vi "Gage-Transfer.vi"(4 "Length (4096)":dbl=4096.0, 5 "Start (0)":dbl, 6 "Segment (1)":u32=1, 7 "Mode (0)":u32 step=1, 8 "Channel (0)":u16 step=1, 9 "Handle Cluster":T1) -> (0 "Error Code":i32, 1 "Actual Length":dbl, 2 "Data in Volts":dbl[](array[numeric]) format="%.2f", 3 "Actual Start":dbl)   [LabVIEW 2022 SP3]
doc: "This VI transfers the data from one channel of the CompuScope system identified by Handle Cluster, which is obtained by calling CsTool-GetSystem.vi. For accurate interpretation of the transferred data, the user should always use the returned Actual Start and Actual Length, and not the requested values. \n\nThis VI can be used for transferring data from 8, 12, 14, and 16 bit CompuScope hardware. Data are transferred from on-board CompuScope memory to PC RAM using PCI Bus Mastering at rates of up to 200 MB/s. \n\nInternally, CsTool-Transfer.vi converts the raw integer ADC code values into double variable voltage values. For more rapid data access, the user may remove the voltage conversion step. The VI will not return programmatic control to LabVIEW until all of the data have been transferred. \n\nIf the call is successful, a 1 is returned in the Error Code indicator. If the call is unsuccessful, an appropriate error code is returned. A descriptive error string may be obtained by calling CsTool-ErrorHandler.vi.\n\n\nInput Value Descriptions:\n\nChannel\nThis integer value specifies the channel from which data are to be transferred. The default value is 0 for the first channel in the CompuScope system. Channels in a LabVIEW CompuScope system begin at 0. If an invalid channel number is given, an error will be returned. Please see the CompuScope hardware manual for more information on channel enumeration.\n\nMode\nThis integer value determines the current transfer mode. Currently, the only valid value for this input is 0.\n\nSegment(1)\nThis integer value determines which Multiple Record segment is to be transferred, if the CompuScope hardware was operating in Multiple Record Mode. For Single Record Mode acquisitions, the user must always set the Record value to 1, which is the default value. If the Record value is too large, an error code will be returned. \n\nStart\nThis double variable value determines the requested starting point of the data transfer from CompuScope memory to PC RAM. Start is specified relative to the trigger address for the acquisition. A Start value of 0 will cause data transfer to begin at the trigger address. Negative Start values are used for the transfer of pre-trigger data. Positive Start values may be used to begin transfer after the trigger address. The default Start value is 0. \n\nLength\nThis double variable value specifies the amount of data, in samples, to be transferred. The default value is 4096. \n\nData in Volts\nThis array variable, of type double, is the LabVIEW buffer variable into which transferred data are returned. The size of the array will be at least Length samples. Data are returned as voltage values, whose conversion depends upon the resolution of the CompuScope system and on the current input range.\n\nActual Start\nThis double variable value returns the actual start point of the data array. The Actual Start may be lower than the requested Start value. This is because the CompuScope memory architecture may force the drivers to download data from an earlier point than the start position. For example, if Start is input to CsTool-Transfer.vi as 0, the Actual Start may return as -2, indicating that two extra samples were returned before the Start position. \n\nThe user must account for the discrepancy between the Start and the Actual Start. The user may choose to ignore samples transferred from before the Start position. Alternatively, the user may conserve these samples, accounting for the fact that the values begin at Actual Start. \n\nActual Length\nThis double variable value returns the actual amount of data transferred, which may be different from the requested Length. The difference, if any, results from CompuScope memory architecture."
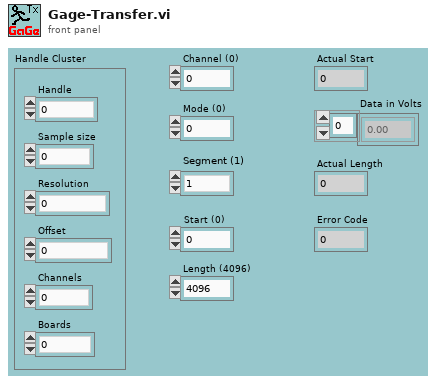
[diagram p1: front panel]
types:
  T1 = cluster{"Handle":u32, "Sample size":u32, "Resolution":i32, "Offset":i32, "Channels":u32, "Boards":u32}
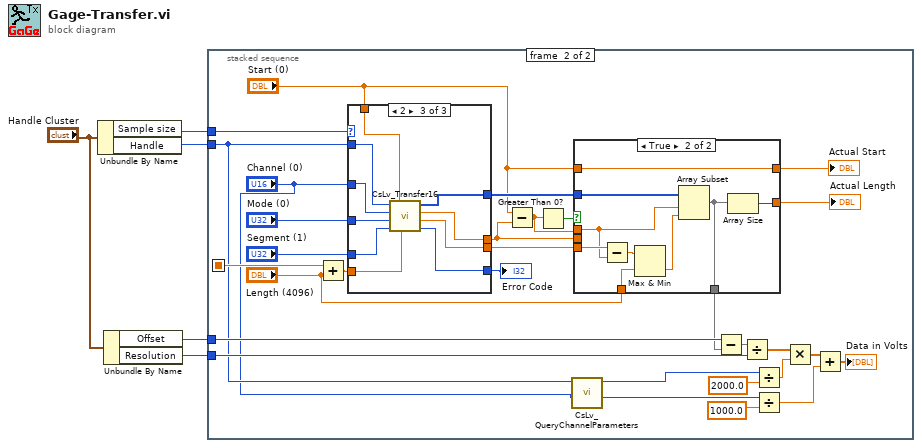
[diagram p0: block diagram]
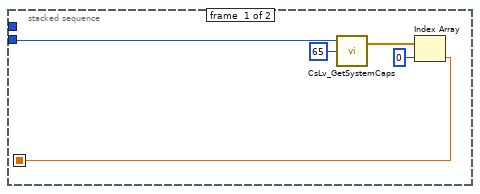
[diagram p2: hidden frame]
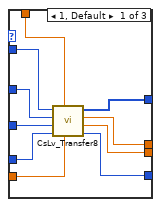
[diagram p4: hidden frame]
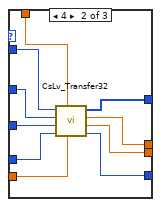
[diagram p5: hidden frame]
diagram:
  n1 = Unbundle By Name("Handle Cluster") -> ("Sample size"=w5:u32, "Handle"=w2:u32)
  n2 = Unbundle By Name("Handle Cluster") -> ("Offset"=w3:i32, "Resolution"=w1:i32)
  n3 = stacked-sequence {
    seq-local: [w6 _] -> [_ w13]
    tunnel: w5 -> [_ w36]
    tunnel: w3 -> [_ w19]
    tunnel: w2 -> [w7 w12]
    tunnel: w1 -> [_ w16]
    frame #0 {
      n4 = call <userlib>:"CsLv_GetSystemCaps.vi"("CapsID"=u16 65, "Handle"=w7) -> ("Buffer"=w9:dbl[])  [unwired: 1 in, 1 out]
      n5 = Index Array(array=w9, index=0) -> (element=w6:dbl)
    }
    frame #1 {
      n6 = Add(x=w13, y="Length (4096)") -> (x+y=w15:dbl)
      n7 = case shown="2" w36 {
        tunnel: w15 -> [w62 w69 w82]
        tunnel: "Segment (1)" -> [w55 w70 w75]
        tunnel: "Mode (0)" -> [w54 w71 w74]
        tunnel: "Start (0)" -> [w61 w68 w81]
        tunnel: [w60 w64 w80] -> w21
        tunnel: [w59 w65 w79] -> w38
        tunnel: [w58 w67 w78] -> w25
        tunnel: w12 -> [w57 w72 w77]
        tunnel: [w56 w66 w76] -> w23
        tunnel: "Channel (0)" -> [w53 w63 w73]
        frame 1, Default {
          n8 = call <userlib>:"CsLv_Transfer8.vi"("Length (4096)"=w62, "Start (0)"=w61, "Segment (1)"=w55, "Mode (0)"=w54, "Channel (0)"=w53, "Handle"=w57) -> ("Error Code"=w59:i32, "Actual Length"=w60:dbl, "Actual Start"=w56:dbl, "Buffer"=w58:u8[])
        }
        frame 4 {
          n9 = call <userlib>:"CsLv_Transfer32.vi"("Length (4096)"=w69, "Start (0)"=w68, "Segment (1)"=w70, "Mode (16)"=w71, "Channel (0)"=w63, "Handle"=w72) -> ("Error Code"=w65:i32, "Actual Length"=w64:dbl, "Actual Start"=w66:dbl, "Buffer"=w67:i32[])
        }
        frame 2 {
          n10 = call <userlib>:"CsLv_Transfer16.vi"("Length (4096)"=w82, "Start (0)"=w81, "Segment (1)"=w75, "Mode (0)"=w74, "Channel (0)"=w73, "Handle"=w77) -> ("Error Code"=w79:i32, "Actual Length"=w80:dbl, "Actual Start"=w76:dbl, "Buffer"=w78:i16[])
        }
      }
      "Error Code" <- w38
      n11 = Subtract(x="Start (0)", y=w23) -> (x-y=w26:dbl)
      n12 = Greater Than 0?(x=w26) -> (x > 0?=w27:bool)
      n13 = call <userlib>:"CsLv_QueryChannelParameters.vi"("Channel"="Channel (0)", "Handle"=w12) -> ("DC Offset (mV)"=w32:i32, "Input Range (mV)"=w31:u32)  [unwired: 5 out]
      n14 = case shown="True" w27 {
        tunnel: w26 -> [_ w49]
        tunnel: [w41 w52] -> w18
        tunnel: w21 -> [w43 w50]
        tunnel: [w43 w51] -> w20
        tunnel: "Length (4096)" -> [_ w46]
        tunnel: w25 -> [w41 w45]
        tunnel: [w42 w44] -> w24
        tunnel: "Start (0)" -> [_ w44]
        tunnel: w23 -> [w42 _]
        frame False {
        }
        frame True {
          n15 = Subtract(x=w50, y=w49) -> (x-y=w48:dbl)
          n16 = Max & Min(x=w48, y=w46) -> (min(x,y)=w47:dbl)  [unwired: 1 out]
          n17 = Array Subset(array=w45, index=w49, length=w47) -> (w52:i32[])
          n18 = Array Size(array=w52) -> (size(s)=w51:i32)
        }
      }
      "Actual Length" <- w20
      "Actual Start" <- w24
      n19 = Subtract(x=w19, y=w18) -> (x-y=w37:i32[])
      n20 = Divide(x=w37, y=w16) -> (x/y=w30:dbl[])
      n21 = Divide(x=w31, y=2000.0) -> (x/y=w29:dbl)
      n22 = Divide(x=w32, y=1000.0) -> (x/y=w28:dbl)
      n23 = Multiply(x=w30, y=w29) -> (x*y=w34:dbl[])
      n24 = Add(x=w34, y=w28) -> (x+y=→"Data in Volts":dbl[])
    }
  }
